vi "SendMessageBack.vi"(2 "CmdArray":string[](array[string])=["aaa"], 3 "receiver process":string[](array[string])=["Return"], 4 "receiver host":string="169.254.8.92", 5 "receiver port (0)":u16=6674) -> (0 "error out":errorcluster, 1 "write time (ms)":u32[](array[numeric])=[1, 0, 0])   [LabVIEW 2018]
uses:
  <vilib>/NI/AMC/Create Single Message.vi
  <vilib>/NI/AMC/Update Message Routing Info.vi
  <vilib>/NI/AMC/Send Message.vi
  <vilib>/NI/AMC/AMC.lvlib
panel:
  in  "message name":string="named"
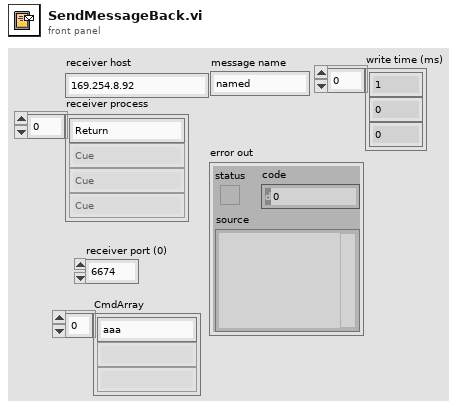
[diagram p1: front panel]
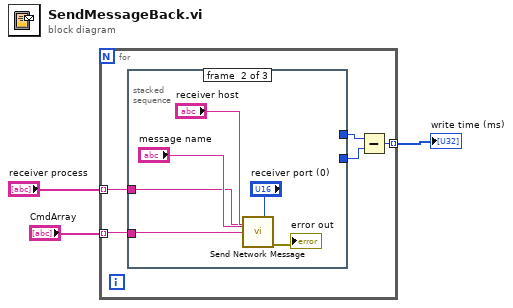
[diagram p0: block diagram]
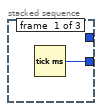
[diagram p2: hidden frame]
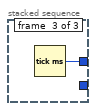
[diagram p3: hidden frame]
diagram:
  n1 = for {
    tunnel: [w6] -> w3 mode=indexing
    tunnel: "receiver process" -> [w5] mode=indexing
    tunnel: "CmdArray" -> [w4] mode=indexing
    n2 = stacked-sequence {
      tunnel: [w9 _ _] -> w7
      tunnel: [_ _ w16] -> w8
      tunnel: w5 -> [_ w12 _]
      tunnel: w4 -> [_ w11 _]
      frame #0 {
        n3 = Tick Count (ms)() -> (millisecond timer value=w9:u32)
      }
      frame #1 {
        n4 = call <vilib>:"Send Network Message.vi"("receiver process"=w12, "receiver host"="receiver host", "receiver port (0)"="receiver port (0)", "message name"="message name", "message value"=w11) -> ("error out"=→"error out":errorcluster)  [unwired: 8 in, 2 out]
      }
      frame #2 {
        n5 = Tick Count (ms)() -> (millisecond timer value=w16:u32)
      }
    }
    n6 = Subtract(x=w8, y=w7) -> (x-y=w6:u32)
  }
  "write time (ms)" <- w3
